vi "Generate Measurement Command.vi"(11 "Measurement Parameters":T2={"Start Step"=0, "End Step"=768, "Cluster Count"=1, "Scan Interval"=1, "Number of Scans"=1, "Measurement Type"=enum."MS"}) -> (3 "Measurement Command":string)   [LabVIEW 2016]
doc: "Creates a URG-04LX compatible string command used to specify the format of an acquisition."
uses:
  Type Definitions/Controls/Measurement Type.ctl
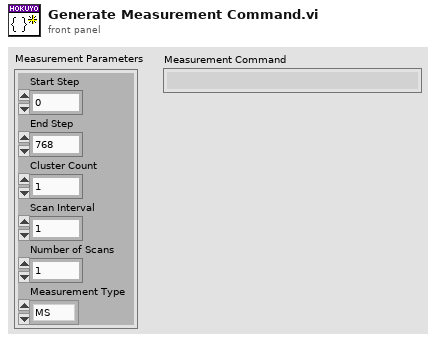
[diagram p1: front panel]
types:
  T1 = typedef "Measurement Type.ctl" = enum16{"MS"}
  T2 = cluster{"Start Step":u32, "End Step":u32, "Cluster Count":u32, "Scan Interval":u32, "Number of Scans":u32, "Measurement Type":T1}
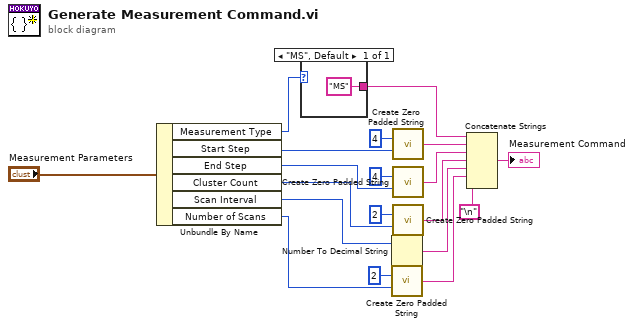
[diagram p0: block diagram]
diagram:
  n1 = Unbundle By Name("Measurement Parameters") -> ("Measurement Type"=w3:T1, "Start Step"=w8:u32, "End Step"=w7:u32, "Cluster Count"=w6:u32, "Scan Interval"=w5:u32, "Number of Scans"=w4:u32)
  n2 = case shown="\"MS\", Default" w3 {
    tunnel: ["MS"] -> w2
    frame "MS", Default {
    }
  }
  n3 = Number To Decimal String(number=w5) -> (decimal integer string=w17:string)  [unwired: 1 in]
  n4 = call "Create Zero Padded String.vi"("Width"=2, "Value"=w4) -> ("Zero Padded Value"=w18:string)  [unwired: 13 in]
  n5 = call "Create Zero Padded String.vi"("Width"=4, "Value"=w8) -> ("Zero Padded Value"=w13:string)  [unwired: 13 in]
  n6 = call "Create Zero Padded String.vi"("Width"=4, "Value"=w7) -> ("Zero Padded Value"=w14:string)  [unwired: 13 in]
  n7 = call "Create Zero Padded String.vi"("Width"=2, "Value"=w6) -> ("Zero Padded Value"=w15:string)  [unwired: 13 in]
  n8 = Concatenate Strings(w2, w13, w14, w15, w17, w18, "\n") -> (→"Measurement Command":string)
